vi "Large integer U8 array - pad shorter.vi"(3 "Large number -U8 2":T1, 5 "Large number -U8 1":T1) -> (0 "Large number -U8 2 out":T1, 2 "Large number -U8 1 out":T1)   [LabVIEW 2012]
doc: "Compares the lengths of the 2 input arrays. The shorter array is padded with 0 elements to make then on equal size.l"
uses:
  User Access Type defs/Large number - U8 array.ctl
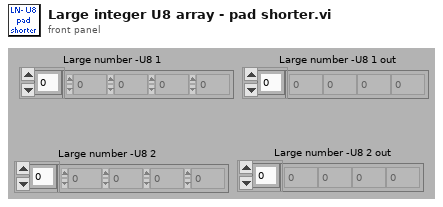
[diagram p1: front panel]
types:
  T1 = typedef "Large number - U8 array.ctl" = u8[]
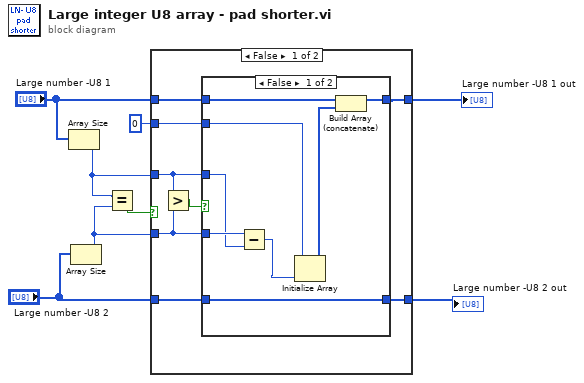
[diagram p0: block diagram]
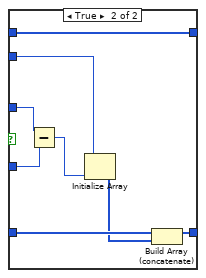
[diagram p2: hidden frame]
diagram:
  n1 = Array Size(array="Large number -U8 1") -> (size(s)=w7:i32)
  n2 = Array Size(array="Large number -U8 2") -> (size(s)=w6:i32)
  n3 = Equal?(x=w7, y=w6) -> (x = y?=w8:bool)
  n4 = case shown="False" w8 {
    tunnel: [w14 w34] -> w3
    tunnel: "Large number -U8 1" -> [w15 w34]
    tunnel: [w12 w33] -> w2
    tunnel: "Large number -U8 2" -> [w13 w33]
    tunnel: w7 -> [w11 _]
    tunnel: w6 -> [w10 _]
    tunnel: u8 0 -> [w9 _]
    frame False {
      n5 = Greater?(x=w11, y=w10) -> (0:w16:bool)
      n6 = case shown="False" w16 {
        tunnel: [w23 w32] -> w14
        tunnel: w15 -> [w24 w32]
        tunnel: w13 -> [w22 w31]
        tunnel: [w22 w30] -> w12
        tunnel: w11 -> [w20 w29]
        tunnel: w10 -> [w21 w28]
        tunnel: w9 -> [w17 w25]
        frame False {
          n7 = Subtract(x=w21, y=w20) -> (x-y=w19:i32)
          n8 = Initialize Array(w17, w19) -> (w18:u8[])
          n9 = Build Array (concatenate)(w24, w18) -> (w23:T1)
        }
        frame True {
          n10 = Subtract(x=w29, y=w28) -> (x-y=w27:i32)
          n11 = Initialize Array(w25, w27) -> (w26:u8[])
          n12 = Build Array (concatenate)(w31, w26) -> (w30:T1)
        }
      }
    }
    frame True {
    }
  }
  "Large number -U8 1 out" <- w3
  "Large number -U8 2 out" <- w2
